vi "SystemClock.vi"() -> (0 "Seconds from Midnight":dbl, 1 "LabVIEW Time Stamp":timestamp, 2 "Output String":string)   [LabVIEW 2022 SP3]
panel:
  out "Minutes":dbl
  out "Hours":dbl
  out "Array":string[](array[string])
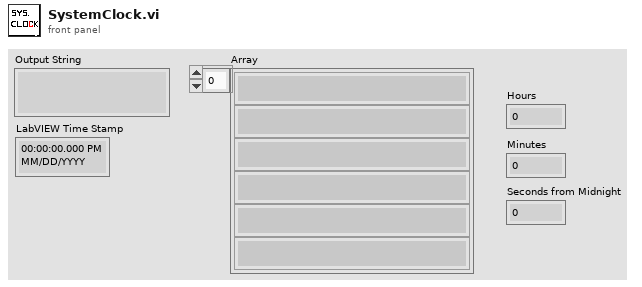
[diagram p1: front panel]
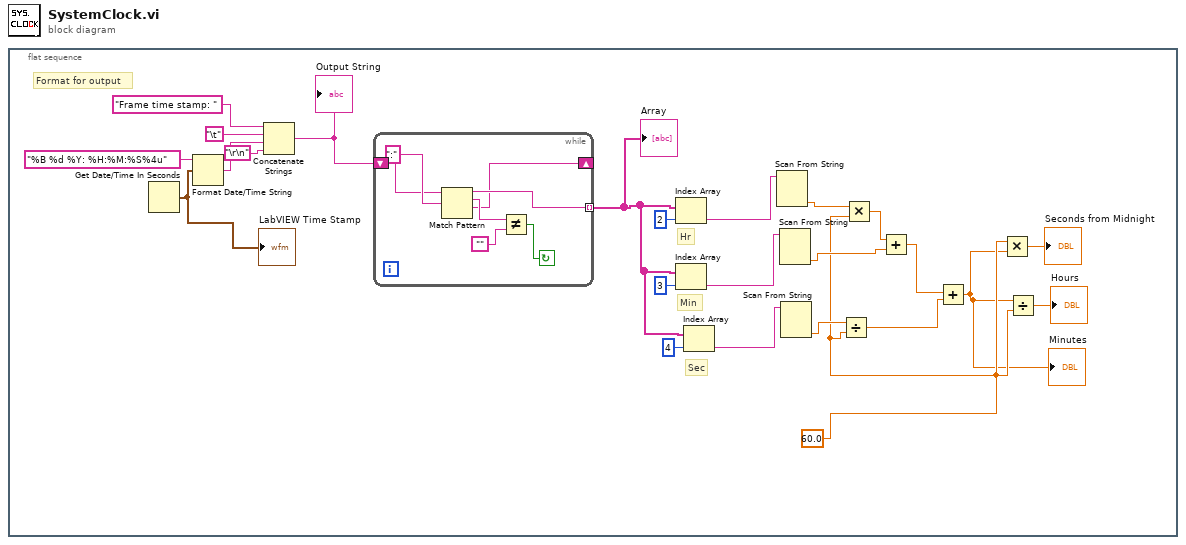
[diagram p0: block diagram]
diagram:
  n1 = flat-sequence {
    frame #0 {
      w3 = 60.0 ("y")
      # "Sec"
      # "Min"
      # "Hr"
      # "Format for output"
      n2 = Get Date/Time In Seconds() -> (seconds since 1Jan1904=w19:timestamp)
      "LabVIEW Time Stamp" <- w19
      n3 = Format Date/Time String(time format string (%c)="%B %d %Y: %H:%M:%S%4u", seconds (now)=w19) -> (date/time string=w24:string)  [unwired: 1 in]
      n4 = Concatenate Strings("Frame time stamp: ", "\t", w24, "\r\n") -> (w18:string)
      "Output String" <- w18
      n5 = while {
        shift-right: [w25] -> _
        shift-left: w18 -> [w27]
        tunnel: [w26] -> w11 mode=indexing
        stop <- w28 continue-if-true
        n6 = Match Pattern(string=w27, regular expression=":") -> (before substring=w26:string, match substring=w30:string, after substring=w25:string)  [unwired: 1 in, 1 out]
        n7 = Not Equal?(x=w30, y="") -> (x != y?=w28:bool)
      }
      "Array" <- w11
      n8 = Index Array(array=w11, index=2) -> (element=w10:string)
      n9 = Index Array(array=w11, index=3) -> (element=w15:string)
      n10 = Index Array(array=w11, index=4) -> (element=w16:string)
      n11 = Scan From String(input string=w10) -> (output 1=w17:dbl)  [unwired: 4 in, 3 out]
      n12 = Scan From String(input string=w15) -> (output 1=w9:dbl)  [unwired: 4 in, 3 out]
      n13 = Scan From String(input string=w16) -> (output 1=w6:dbl)  [unwired: 4 in, 3 out]
      n14 = Divide(x=w6, y=w3) -> (x/y=w5:dbl)
      n15 = Multiply(x=w17, y=w3) -> (x*y=w8:dbl)
      n16 = Add(x=w8, y=w9) -> (x+y=w7:dbl)
      n17 = Add(x=w7, y=w5) -> (x+y=w2:dbl)
      "Minutes" <- w2
      n18 = Multiply(x=w3, y=w2) -> (x*y=→"Seconds from Midnight":dbl)
      n19 = Divide(x=w2, y=w3) -> (x/y=→"Hours":dbl)
    }
  }
